vi "Check if configuration files exist.vi"(8 "error in (no error)":errorcluster, 11 "StageSPIMBase in":refnum<class "StageSPIM.lvclass">) -> (0 "error out":errorcluster, 2 "configuration file exists?":bool, 3 "StageSPIMBase out":refnum<class "StageSPIM.lvclass">)   [LabVIEW 2012, in "StageSPIM.lvclass"]
doc: "Checks whether all required configuration files for the component exist."
uses:
  StageSPIM.lvclass
  <vilib>/Distrio/Murmex/Murmex/Murmex.lvclass
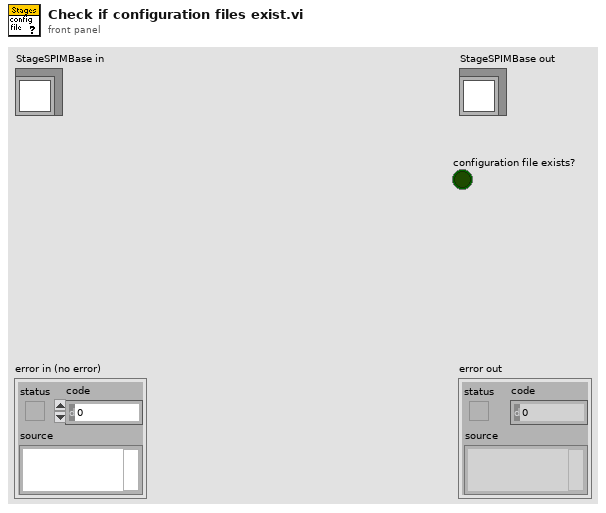
[diagram p1: front panel]
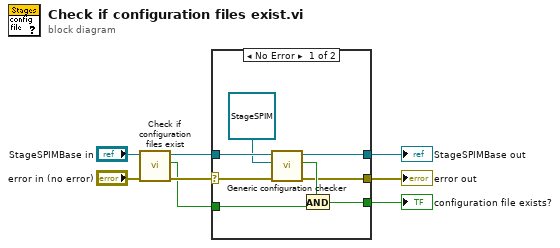
[diagram p0: block diagram]
diagram:
  n1 = call-parent "Check if configuration files exist.vi"("error in (no error)"="error in (no error)", "MurmexBase in"="StageSPIMBase in") -> ("error out"=w6:errorcluster, "configuration file exists?"=w4:bool, "MurmexBase out"=w5:refnum<class "StageSPIM.lvclass">)  [unwired: 7 in]
  n2 = case shown="No Error" w6 {
    selector: w6 -> [w15 w18]
    tunnel: w5 -> [w13 w19]
    tunnel: w4 -> [w10 w17]
    tunnel: [w14 w18] -> w3
    tunnel: [w12 w19] -> w2
    tunnel: [w11 w17] -> w1
    frame No Error {
      n3 = call <vilib>:"Generic configuration checker.vi"("error in (no error)"=w15, "inheritance level"=refnum<class "StageSPIM.lvclass"> refnum ("StageSPIM.lvclass"), "Murmex in"=w13) -> ("error out"=w14:errorcluster, "configuration file exists?"=w16:bool, "Murmex out"=w12:refnum<class "StageSPIM.lvclass">)  [unwired: 6 in]
      n4 = And(x=w16, y=w10) -> (x .and. y?=w11:bool)
    }
    frame Error {
    }
  }
  "error out" <- w3
  "StageSPIMBase out" <- w2
  "configuration file exists?" <- w1
